vi "Bertta_v03.vi"() -> ()   [LabVIEW 2015]
uses:
  BERTTA.dll
panel:
  in  "Tab Control":T1(tab)
  out "Mettler":dynamicdata(graph)
  out "Lauda":dynamicdata(graph)
  in  "col":i32=3
  out "Table":string[][](table)
  in  "col 2":i32=4
  in  "new element/subarray":string[](array[string])
  in  "?":T2(tab)
  out "rc":i32
  in  "Kd":dbl
  in  "Ki":dbl
  in  "Kp":dbl=2.0
  out "PID output":dbl
  in  "Temp setpoint":dbl=20.0
  in  "Device port":dbl=1.0
  out "Debug msg":dbl
  out "Temp Lauda":dbl
  out "Timestep":i32
  in  "Device port":i32=2
  out "Weight":dbl
  out "Weight":dbl
  in  "Device port":i32=6
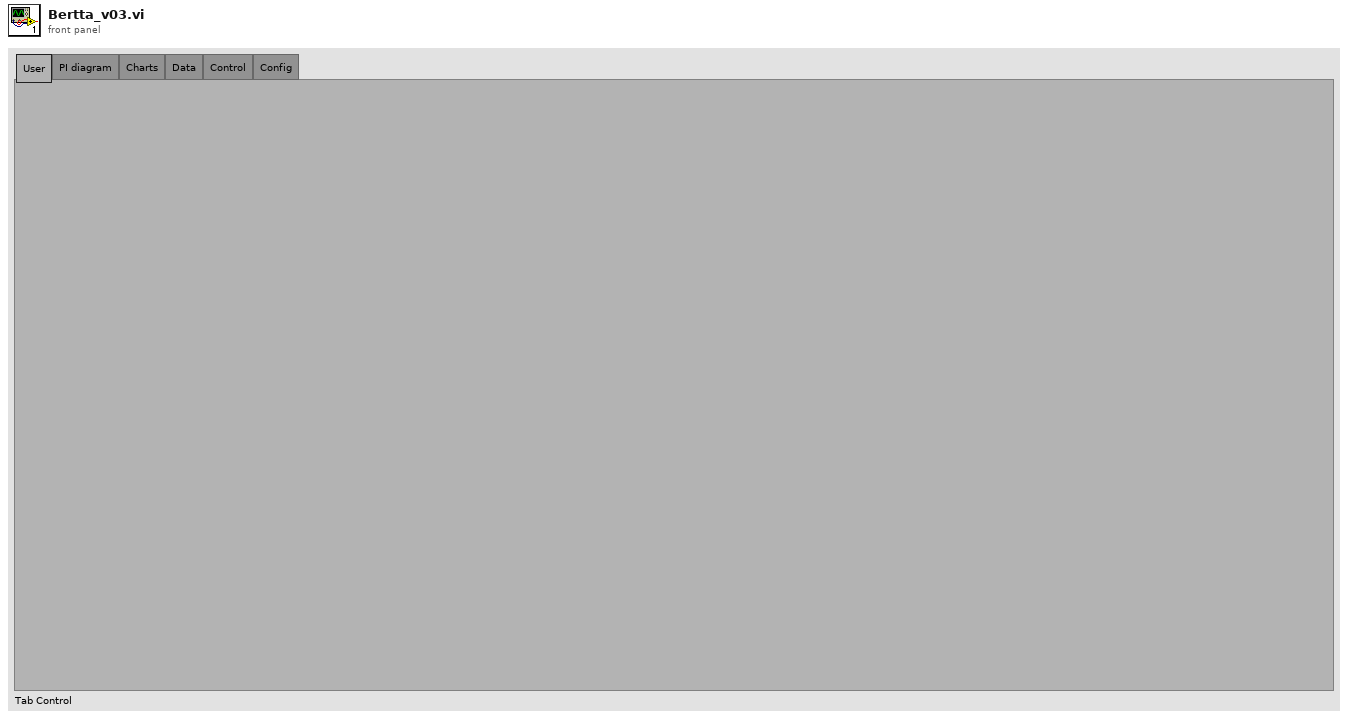
[diagram p1: front panel]
types:
  T1 = enum32{"User", "PI diagram", "Charts", "Data", "Control", "Config"}
  T2 = enum32{"DB / File", "Lauda", "Heidolph", "Mettler 1", "Mettler 2", "Mettler 3"}
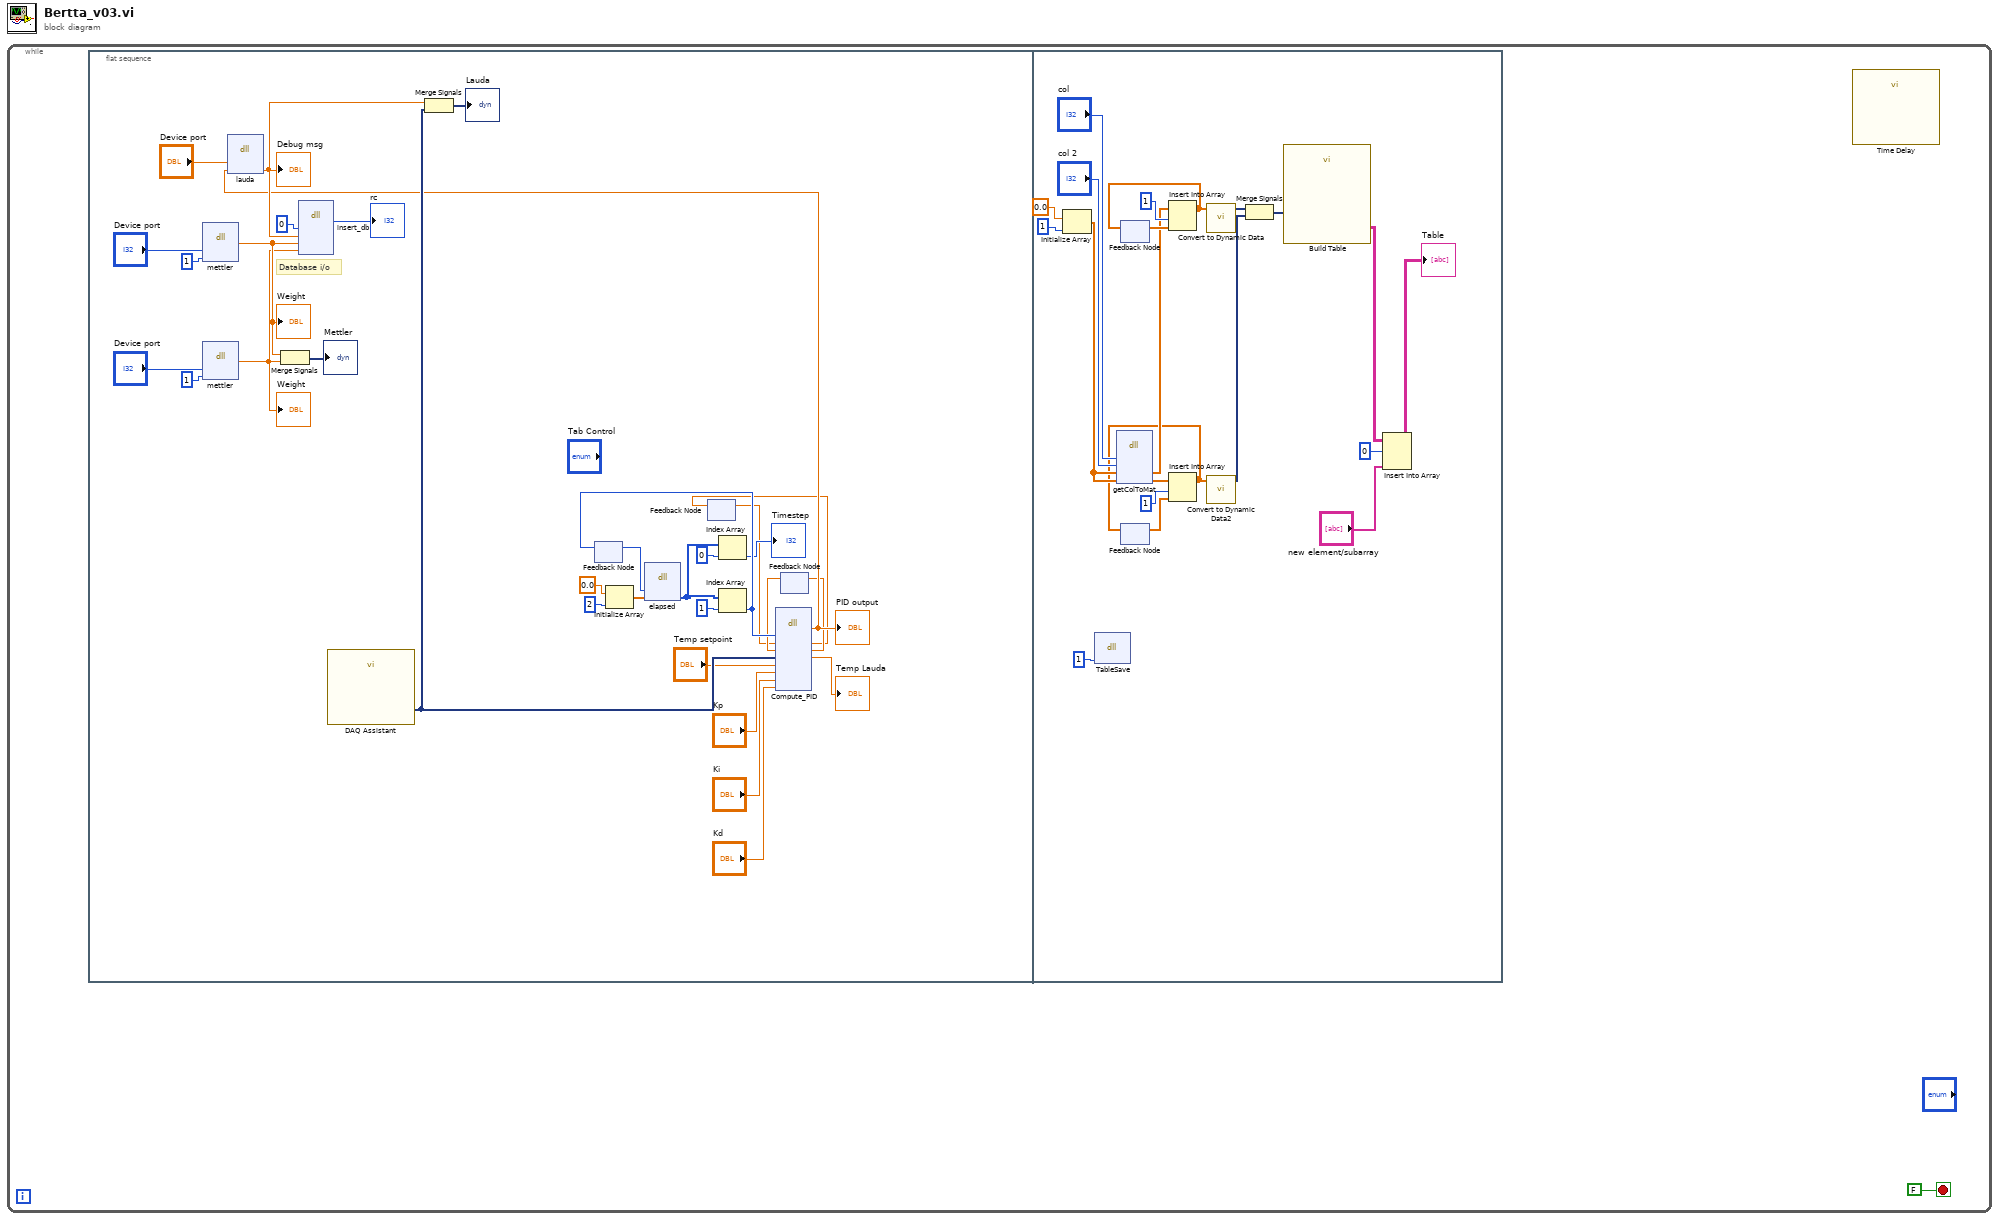
[diagram p0: block diagram]
diagram:
  n1 = while {
    stop <- FALSE stop-if-true
    n2 = flat-sequence {
      frame #0 {
        # "Database i/o"
        n3 = dll-call lib="C:/Users/xlaraser/Documents/Visual Studio 2017/Projects/Bertta/BERTTA/Debug/BERTTA.dll" fn="mettler"("port"="Device port", "msg"=1) -> ("return type"=w17:dbl)  [unwired: 5 in, 2 out]
        "Weight" <- w17
        n4 = dll-call lib="C:/Users/xlaraser/Documents/Visual Studio 2017/Projects/Bertta/BERTTA/Debug/BERTTA.dll" fn="mettler"("port"="Device port", "msg"=1) -> ("return type"=w16:dbl)  [unwired: 5 in, 2 out]
        "Weight" <- w16
        n5 = Merge Signals(w17, w16) -> (→"Mettler":dynamicdata)
        n6 = call "DAQ Assistant"() -> ("data"=w28:dynamicdata)  [unwired: 17 in, 2 out]
        n7 = feedback #1() -> (w14:i32)  [unwired: 1 in]
        n8 = Initialize Array(0.0 ("element"), 2 ("dimension size")) -> (w12:dbl[])
        n9 = dll-call lib="C:/Users/xlaraser/Documents/Visual Studio 2017/Projects/Bertta/BERTTA/Debug/BERTTA.dll" fn="elapsed"("last_time"=w14, "params"=w12) -> ("params"=w9:i32[])  [unwired: 5 in, 2 out]
        n10 = feedback #2() -> (w4:dbl)  [unwired: 1 in]
        n11 = Index Array(array=w9, index=0) -> (element=→"Timestep":i32)
        n12 = Index Array(array=w9, index=1) -> (element=w10:i32)
        n13 = feedback-in #1(w10) -> ()
        n14 = feedback #3() -> (w6:dbl)  [unwired: 1 in]
        n15 = dll-call lib="C:/Users/xlaraser/Documents/Visual Studio 2017/Projects/Bertta/BERTTA/Debug/BERTTA.dll" fn="Compute_PID"("timeChange"=w10, "errSum"=w4, "lastErr"=w6, "Input"=w28, "Setpoint"="Temp setpoint", "kp"="Kp", "ki"="Ki", "kd"="Kd") -> ("return type"=w26:dbl, "errSum"=w5:dbl, "lastErr"=w7:dbl, "Input"=→"Temp Lauda":dbl)  [unwired: 8 in, 2 out]
        "PID output" <- w26
        n16 = dll-call lib="C:/Users/xlaraser/Documents/Visual Studio 2017/Projects/Bertta/BERTTA/Debug/BERTTA.dll" fn="lauda"("port"="Device port", "set_temp"=w26) -> ("set_temp"=w30:dbl)  [unwired: 5 in, 2 out]
        "Debug msg" <- w30
        n17 = dll-call lib="C:/Users/xlaraser/Documents/Visual Studio 2017/Projects/Bertta/BERTTA/Debug/BERTTA.dll" fn="insert_db"("heidolph"=0, "lauda"=w30, "mettler1"=w17, "mettler2"=w16) -> ("return type"=→"rc":i32)  [unwired: 7 in, 2 out]
        n18 = Merge Signals(w30, w28) -> (→"Lauda":dynamicdata)
        n19 = feedback-in #2(w5) -> ()
        n20 = feedback-in #3(w7) -> ()
      }
      frame #1 {
        n21 = Initialize Array(0.0 ("element"), 1 ("dimension size")) -> (w50:dbl[])
        n22 = dll-call lib="C:/Users/xlaraser/Documents/Visual Studio 2017/Projects/Bertta/BERTTA/Debug/BERTTA.dll" fn="TableSave"("exec"=1) -> ()  [unwired: 5 in, 2 out]
        n23 = dll-call lib="C:/Users/xlaraser/Documents/Visual Studio 2017/Projects/Bertta/BERTTA/Debug/BERTTA.dll" fn="getColToMat"("col1"="col", "col2"="col 2", "values1"=w50, "values2"=w50) -> ("values1"=w36:dbl[], "values2"=w42:dbl[])  [unwired: 6 in, 2 out]
        n24 = feedback #4() -> (w38:dbl[])  [unwired: 1 in]
        n25 = feedback #5() -> (w41:dbl[])  [unwired: 1 in]
        n26 = Insert Into Array(array=w36, index=1, new element=w38) -> (w35:dbl[])
        n27 = feedback-in #4(w35) -> ()
        n28 = Insert Into Array(array=w42, index=1, new element=w41) -> (w34:dbl[])
        n29 = feedback-in #5(w34) -> ()
        n30 = call "Convert to Dynamic Data"("Array"=w35) -> ("Dynamic Data Type"=w48:dynamicdata)  [unwired: 3 in]
        n31 = call "Convert to Dynamic Data2"("Array"=w34) -> ("Dynamic Data Type"=w47:dynamicdata)  [unwired: 3 in]
        n32 = Merge Signals(w48, w47) -> (w46:dynamicdata)
        n33 = call "Build Table"("Signals"=w46) -> ("Table"=w39:string[][])  [unwired: 4 in, 6 out]
        n34 = Insert Into Array(array=w39, index (row)=0, new element="new element/subarray") -> (→"Table":string[][])  [unwired: 1 in]
      }
    }
    n35 = call "Time Delay"() -> ()  [unwired: 11 in, 1 out]
  }
